vi "字符串精度转换.vi"(9 "数组输入":string[](array[string]), 11 "输入字符串":string) -> (1 "数组输出":string[](array[string]), 3 "输出字符串":string)   [LabVIEW 2016, in "数据传输系统.lvlib"]
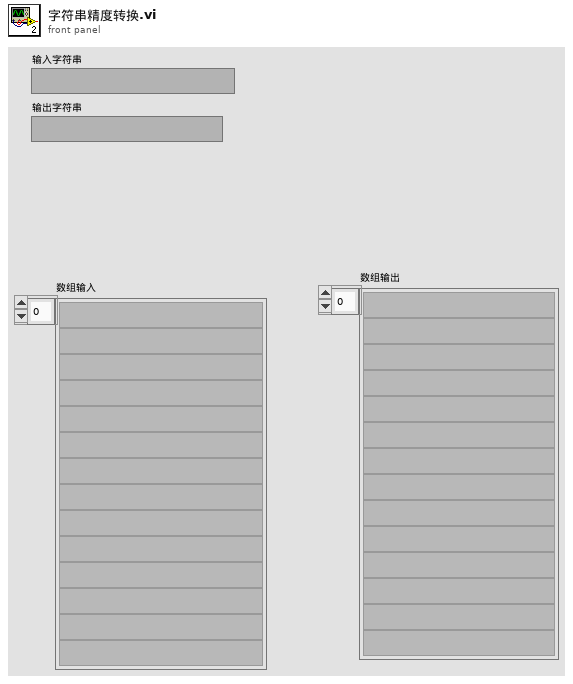
[diagram p1: front panel]
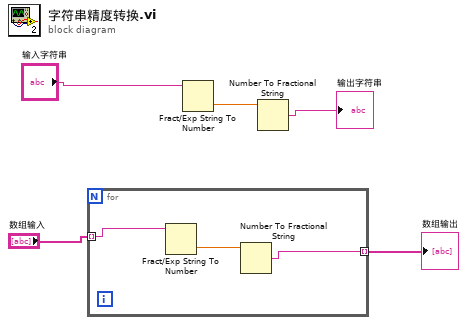
[diagram p0: block diagram]
diagram:
  n1 = for {
    tunnel: "数组输入" -> [w7] mode=indexing
    tunnel: [w6] -> w1 mode=indexing
    n2 = Fract/Exp String To Number(string=w7) -> (number=w8:dbl)  [unwired: 3 in, 1 out]
    n3 = Number To Fractional String(number=w8) -> (F-format string=w6:string)  [unwired: 3 in]
  }
  "数组输出" <- w1
  n4 = Fract/Exp String To Number(string="输入字符串") -> (number=w5:dbl)  [unwired: 3 in, 1 out]
  n5 = Number To Fractional String(number=w5) -> (F-format string=→"输出字符串":string)  [unwired: 3 in]
